vi "Multiple Nano-Drives Information.vi"() -> ()   [LabVIEW 2012]
uses:
  Madlib.dll
panel:
  in  "Case Constant\n(See Context Help)":bool=TRUE
  out "Serial #":i32
  in  "Release Handles":bool
  out "Aux Calibration":dbl format="%.3f"
  out "Z Calibration":dbl format="%.3f"
  out "Y Calibration":dbl format="%.3f"
  out "X Calibration":dbl caption="Calibration (um)" format="%.3f"
  out "Aux axis":bool
  out "Z axis":bool
  out "Y axis":bool
  out "X axis":bool
  out "DAC Freq (ms)":dbl format="%.4f"
  out "ADC Freq (ms)":dbl format="%.4f"
  out "Dll Revision":i16
  out "Dll Version":i16
  out "ADC resolution (bits)":i16
  out "DAC resolution (bits)":i16
  out "Product ID (in hex)":string
  out "Firmware Version":i16
  out "Firmware Profile":i16
  in  "Tab Control":T1(tab)
  out "Handle":i32
  out "Handle 2":i32 caption="Handle"
  out "Handle 3":i32 caption="Handle"
  out "Handle 4":i32 caption="Handle"
  out "Handle 5":i32 caption="Handle"
  # "Provides information about all of the Nano-Drives attached."
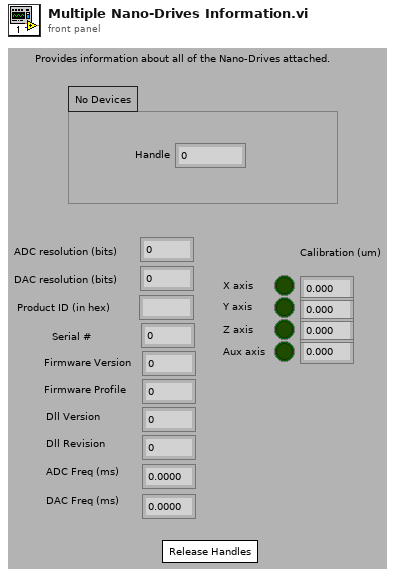
[diagram p1: front panel]
types:
  T1 = enum32{"Page 1", "Page 2", "Page 3", "Page 4", "Page 5"}
  T2 = cluster{i32, i32, string, i32, i32, bool, bool, bool, bool, dbl, dbl, dbl, dbl, i32, i32, dbl, dbl, i32}
  T3 = cluster{i32, i32, string, i32, i32, bool, bool, bool, bool, dbl, dbl, dbl, dbl, i32, i32, dbl, dbl, i32}[]
  T4 = cluster{"ADC resolution (bits)":i16, "DAC resolution (bits)":i16, "Product ID (in hex)":string, "Firmware Version":i16, "Firmware Profile":i16, "X axis":bool, "Y axis":bool, "Z axis":bool, "Aux axis":bool, "X Calibration":dbl, "Y Calibration":dbl, "Z Calibration":dbl, "Aux Calibration":dbl, "Dll Version":i16, "Dll Revision":i16, "ADC Freq (ms)":dbl, "DAC Freq (ms)":dbl, "Serial #":i32}
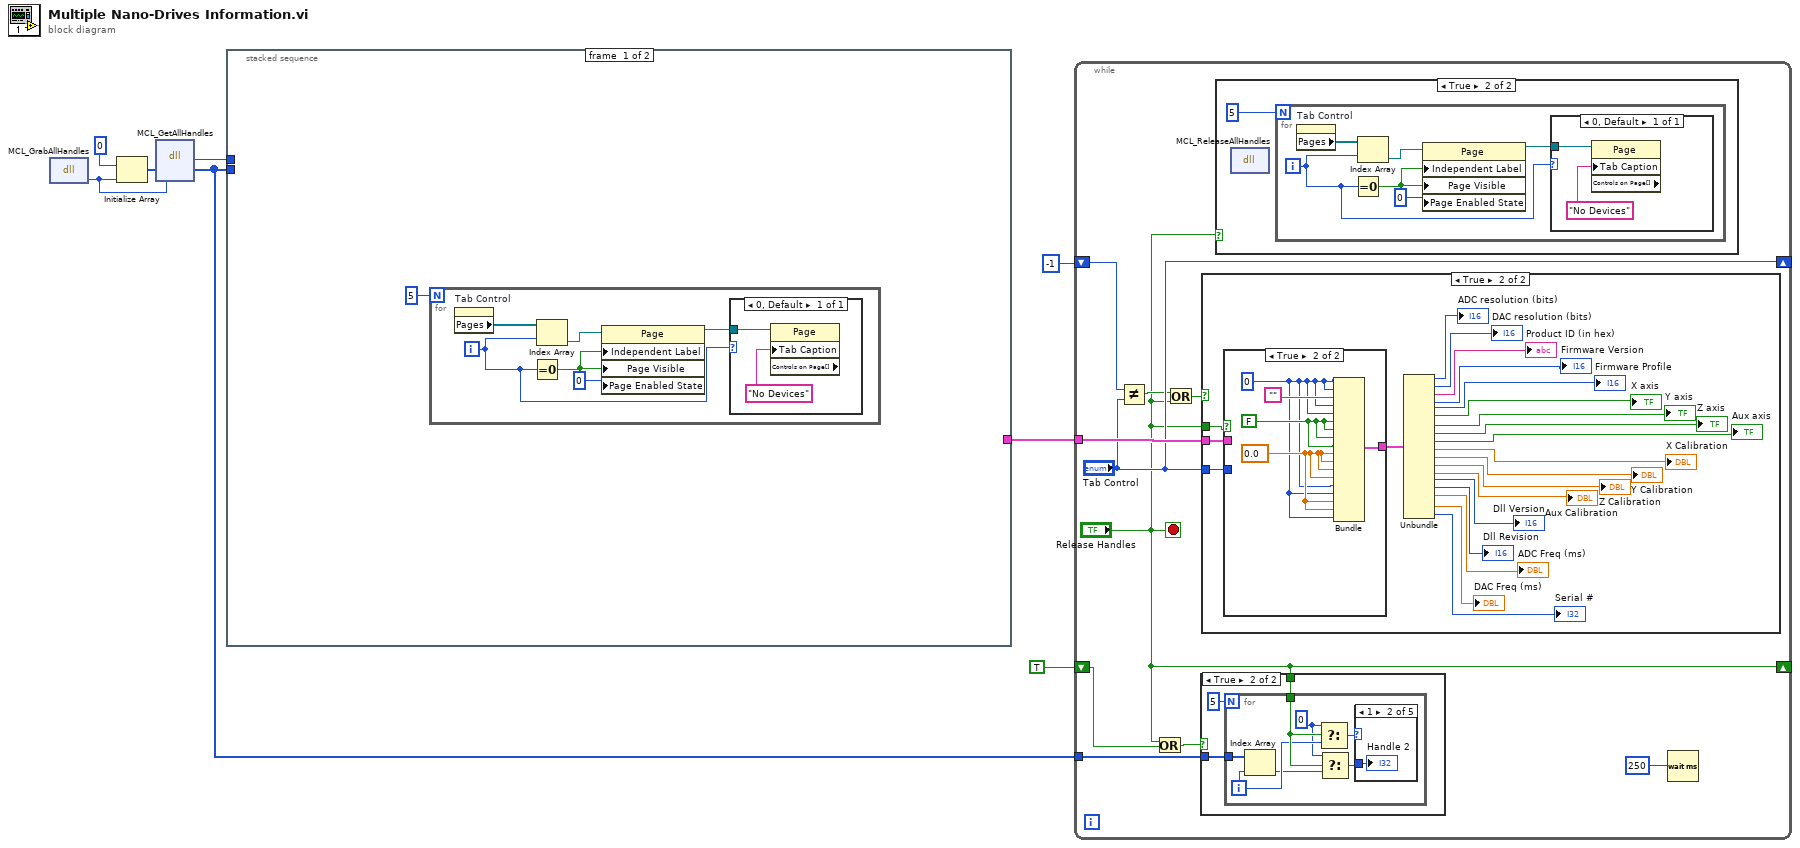
[diagram p0: block diagram]
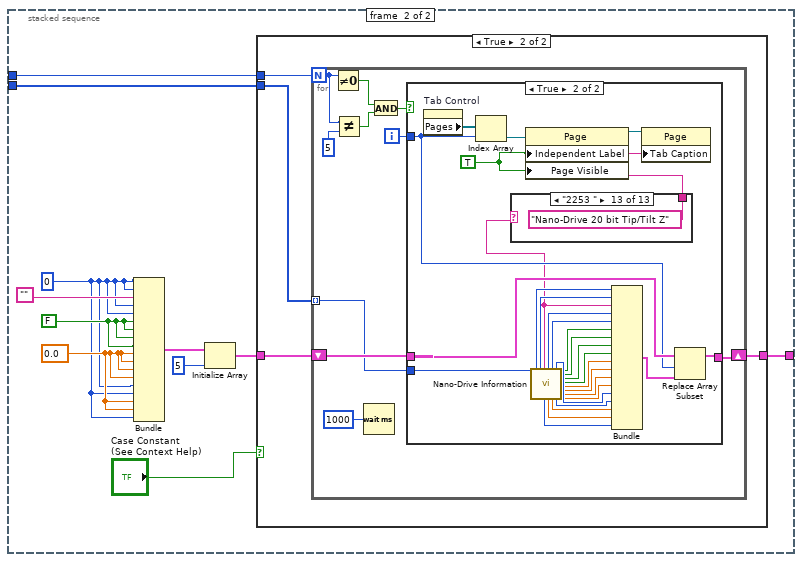
[diagram p2: hidden frame]
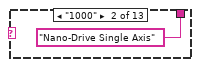
[diagram p6: hidden frame]
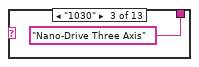
[diagram p7: hidden frame]
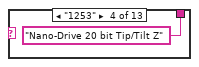
[diagram p8: hidden frame]
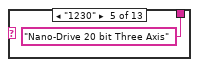
[diagram p9: hidden frame]
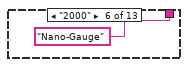
[diagram p10: hidden frame]
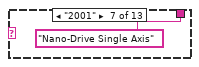
[diagram p11: hidden frame]
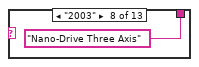
[diagram p12: hidden frame]
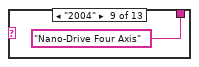
[diagram p13: hidden frame]
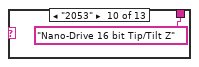
[diagram p14: hidden frame]
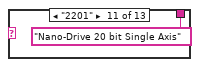
[diagram p15: hidden frame]
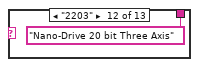
[diagram p16: hidden frame]
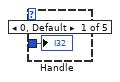
[diagram p18: hidden frame]
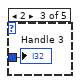
[diagram p19: hidden frame]
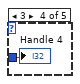
[diagram p20: hidden frame]
diagram:
  n1 = dll-call lib="C:/Users/Labview/Desktop/SRR/Madlib_x64/Labview Examples/MADLib.dll" fn="MCL_GrabAllHandles"() -> (w3:i32)  [unwired: 3 in, 2 out]
  n2 = Initialize Array(0, w3) -> (w4:i32[])
  n3 = dll-call lib="C:/Users/Labview/Desktop/SRR/Madlib_x64/Labview Examples/MADLib.dll" fn="MCL_GetAllHandles"("handles"=w4, "size"=w3) -> (w2:i32, "handles"=w1:i32[])  [unwired: 4 in, 2 out]
  n4 = stacked-sequence {
    tunnel: [_ w22] -> w8
    tunnel: w2 -> [_ w19]
    tunnel: w1 -> [_ w18]
    frame #0 {
      n5 = for {
        N: 5 -> [_]
        i -> [w10]
        n6 = property on="Tab Control" class="TabCtl (strict)"() -> ("Pages"=w15:refnum<vi>[])  [unwired: 2 in, 2 out]
        n7 = Equal To 0?(x=w10) -> (x = 0?=w12:bool)
        n8 = Index Array(array=w15, index=w10) -> (element=w14:refnum<vi>)
        n9 = property class="Page"(reference=w14, "Independent Label"=w12, "Page Visible"=w12, "Page Enabled State"=0) -> (reference out=w13:refnum<vi>)  [unwired: 1 in, 1 out]
        n10 = case shown="0, Default" w10 {
          tunnel: w13 -> [w17]
          frame 0, Default {
            n11 = property class="Page" props=["Tab Caption", "Controls on Page[]"](reference=w17, "Tab Caption"="No Devices") -> ()  [unwired: 1 in, 3 out]
          }
        }
      }
    }
    frame #1 {
      w21 = FALSE
      w24 = 0.0
      w20 = 0
      n12 = Bundle(w20, w20, "", w20, w20, w21, w21, w21, w21, w24, w24, w24, w24, w20, w20, w24, w24, w20) -> (w27:T2)  [unwired: 1 in]
      n13 = Initialize Array(w27, 5) -> (w26:T3)
      n14 = case shown="True" "Case Constant\n(See Context Help)" {
        tunnel: [_ w32] -> w22
        tunnel: w26 -> [_ w31]
        tunnel: w19 -> [_ w30]
        tunnel: w18 -> [_ w29]
        frame False {
        }
        frame True {
          n15 = for {
            N: w30 -> [w37]
            shift-right: [w41] -> w32
            shift-left: w31 -> [w40]
            tunnel: w29 -> [w38] mode=indexing
            i -> [w39]
            n16 = Not Equal To 0?(x=w37) -> (x != 0?=w34:bool)
            n17 = Not Equal?(x=w37, y=5) -> (x != y?=w33:bool)
            n18 = Wait (ms)(milliseconds to wait=1000) -> ()  [unwired: 1 out]
            n19 = And(x=w34, y=w33) -> (x .and. y?=w35:bool)
            n20 = case shown="True" w35 {
              tunnel: w38 -> [_ w55]
              tunnel: [w43 w54] -> w41
              tunnel: w40 -> [w43 w53]
              tunnel: w39 -> [_ w47]
              frame False {
              }
              frame True {
                w48 = TRUE
                n21 = property on="Tab Control" class="TabCtl (strict)"() -> ("Pages"=w51:refnum<vi>[])  [unwired: 2 in, 2 out]
                n22 = Index Array(array=w51, index=w47) -> (element=w50:refnum<vi>)
                n23 = property class="Page"(reference=w50, "Independent Label"=w48, "Page Visible"=w48) -> (reference out=w49:refnum<vi>)  [unwired: 1 in, 1 out]
                n24 = call "Nano-Drive Information.vi"("Handle"=w55) -> ("ADC resolution (bits)"=w56:i16, "DAC resolution (bits)"=w57:i16, "Product ID (in hex)"=w45:string, "Serial #"=w46:i32, "Firmware Version"=w58:i16, "DAC Freq (ms)"=w71:dbl, "Firmware Profile"=w59:i16, "ADC Freq (ms)"=w70:dbl, "Dll Version"=w68:i16, "Dll Revision"=w69:i16, "X axis"=w60:bool, "Y axis"=w61:bool, "Z axis"=w62:bool, "Aux axis"=w63:bool, "X Calibration"=w64:dbl, "Y Calibration"=w65:dbl, "Z Calibration"=w66:dbl, "Aux Calibration"=w67:dbl)  [unwired: 9 in]
                n25 = case shown="\"2253 \"" w45 {
                  selector: w45 -> [w72 _ _ _ _ _ _ _ _ _ _ _ _]
                  tunnel: [w72 "Nano-Drive Single Axis" "Nano-Drive Three Axis" "Nano-Drive 20 bit Tip/Tilt Z" "Nano-Drive 20 bit Three Axis" "Nano-Gauge" "Nano-Drive Single Axis" "Nano-Drive Three Axis" "Nano-Drive Four Axis" "Nano-Drive 16 bit Tip/Tilt Z" "Nano-Drive 20 bit Single Axis" "Nano-Drive 20 bit Three Axis" "Nano-Drive 20 bit Tip/Tilt Z"] -> w44
                  frame "", Default {
                  }
                  frame "1000" {
                  }
                  frame "1030" {
                  }
                  frame "1253" {
                  }
                  frame "1230" {
                  }
                  frame "2000" {
                  }
                  frame "2001" {
                  }
                  frame "2003" {
                  }
                  frame "2004" {
                  }
                  frame "2053" {
                  }
                  frame "2201" {
                  }
                  frame "2203" {
                  }
                  frame "2253 " {
                  }
                }
                n26 = Bundle("ADC resolution (bits)"=w56, "DAC resolution (bits)"=w57, "Product ID (in hex)"=w45, "Firmware Version"=w58, "Firmware Profile"=w59, "X axis"=w60, "Y axis"=w61, "Z axis"=w62, "Aux axis"=w63, "X Calibration"=w64, "Y Calibration"=w65, "Z Calibration"=w66, "Aux Calibration"=w67, "Dll Version"=w68, "Dll Revision"=w69, "ADC Freq (ms)"=w70, "DAC Freq (ms)"=w71, "Serial #"=w46) -> (w52:T4)  [unwired: 1 in]
                n27 = property class="Page"(reference=w49, "Tab Caption"=w44) -> ()  [unwired: 1 in, 2 out]
                n28 = Replace Array Subset(array=w53, new element=w52, index=w47) -> (w54:T3)
              }
            }
          }
        }
      }
    }
  }
  n29 = while {
    tunnel: w8 -> [w94]
    tunnel: w1 -> [w93]
    shift-right: ["Tab Control"] -> _
    shift-left: -1 -> [w91]
    shift-right: ["Release Handles"] -> _
    shift-left: TRUE -> [w86]
    stop <- "Release Handles" stop-if-true
    n30 = Not Equal?(x=w91, y="Tab Control") -> (x != y?=w89:bool)
    n31 = Or(x="Release Handles", y=w86) -> (x .or. y?=w88:bool)
    n32 = Or(x=w89, y="Release Handles") -> (x .or. y?=w90:bool)
    n33 = case shown="True" w88 {
      tunnel: w93 -> [_ w96]
      tunnel: "Release Handles" -> [_ w95]
      frame False {
      }
      frame True {
        n34 = for {
          N: 5 -> [_]
          tunnel: w96 -> [w104]
          tunnel: w95 -> [w101]
          i -> [w100]
          w98 = 0
          n35 = Index Array(array=w104, index=w100) -> (element=w99:i32)
          n36 = Select(t=w98, s=w101, f=w100) -> (s? t:f=w103:i32)
          n37 = Select(t=w98, s=w101, f=w99) -> (s? t:f=w102:i32)
          n38 = case shown="1" w103 {
            tunnel: w102 -> [w105 w106 w107 w108 w109]
            frame 0, Default {
              "Handle" <- w105
            }
            frame 1 {
              "Handle 2" <- w106
            }
            frame 2 {
              "Handle 3" <- w107
            }
            frame 3 {
              "Handle 4" <- w108
            }
            frame 4 {
              "Handle 5" <- w109
            }
          }
        }
      }
    }
    n39 = case shown="True" w90 {
      tunnel: w94 -> [_ w130]
      tunnel: "Tab Control" -> [_ w112]
      tunnel: "Release Handles" -> [_ w111]
      frame False {
      }
      frame True {
        n40 = case shown="True" w111 {
          tunnel: w130 -> [w134 _]
          tunnel: [w133 w137] -> w129
          tunnel: w112 -> [w132 _]
          frame False {
            n41 = Index Array(array=w134, index=w132) -> (element=w133:T2)
          }
          frame True {
            w135 = 0
            w138 = 0.0
            w136 = FALSE
            n42 = Bundle(w135, w135, "", w135, w135, w136, w136, w136, w136, w138, w138, w138, w138, w135, w135, w138, w138, w135) -> (w137:T2)  [unwired: 1 in]
          }
        }
        n43 = Unbundle(w129) -> (→"ADC resolution (bits)":i32, →"DAC resolution (bits)":i32, →"Product ID (in hex)":string, →"Firmware Version":i32, →"Firmware Profile":i32, →"X axis":bool, →"Y axis":bool, →"Z axis":bool, →"Aux axis":bool, →"X Calibration":dbl, →"Y Calibration":dbl, →"Z Calibration":dbl, →"Aux Calibration":dbl, →"Dll Version":i32, →"Dll Revision":i32, →"ADC Freq (ms)":dbl, →"DAC Freq (ms)":dbl, →"Serial #":i32)
      }
    }
    n44 = case shown="True" "Release Handles" {
      frame False {
      }
      frame True {
        n45 = dll-call lib="C:/Users/Labview/Desktop/SRR/Madlib_x64/Labview Examples/MADLib.dll" fn="MCL_ReleaseAllHandles"() -> ()  [unwired: 4 in, 2 out]
        n46 = for {
          N: 5 -> [_]
          i -> [w141]
          n47 = property on="Tab Control" class="TabCtl (strict)"() -> ("Pages"=w146:refnum<vi>[])  [unwired: 2 in, 2 out]
          n48 = Equal To 0?(x=w141) -> (x = 0?=w143:bool)
          n49 = Index Array(array=w146, index=w141) -> (element=w145:refnum<vi>)
          n50 = property class="Page"(reference=w145, "Independent Label"=w143, "Page Visible"=w143, "Page Enabled State"=0) -> (reference out=w144:refnum<vi>)  [unwired: 1 in, 1 out]
          n51 = case shown="0, Default" w141 {
            tunnel: w144 -> [w148]
            frame 0, Default {
              n52 = property class="Page" props=["Tab Caption", "Controls on Page[]"](reference=w148, "Tab Caption"="No Devices") -> ()  [unwired: 1 in, 3 out]
            }
          }
        }
      }
    }
    n53 = Wait (ms)(milliseconds to wait=250) -> ()  [unwired: 1 out]
  }
